vi "SJ_Enter_Data.vi"() -> (3 "SJ Data OUT":T1={"Do (mm)"=3.0, "Dc (mm)"=0.039, "Ho (mm)"=0.01, "Hc (mm)"=0.006, "K"=1.251, "beta"=1.039, "Vc (m^3)"=0.0, "Vo (m^3)"=0.0})   [LabVIEW 2011]
uses:
  Controls/SJ_Data_Cluster.ctl
panel:
  out "String":string
  in  "OK Button":bool
  in  "SJ Data IN":T1={"Do (mm)"=3.0, "Dc (mm)"=0.039, "Ho (mm)"=0.01, "Hc (mm)"=0.006, "K"=1.251, "beta"=1.039, "Vc (m^3)"=0.0, "Vo (m^3)"=0.0}
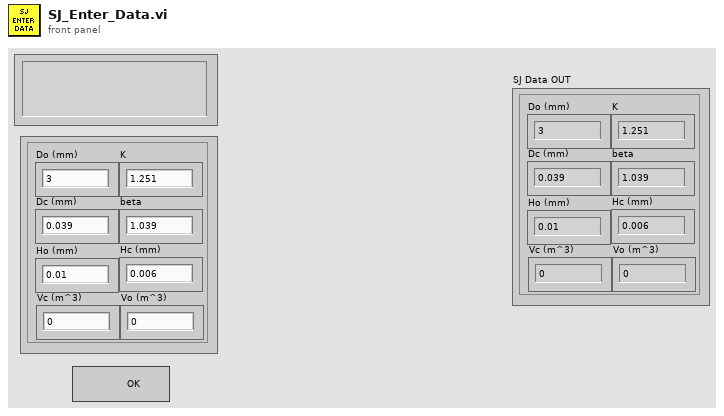
[diagram p1: front panel]
types:
  T1 = typedef "SJ_Data_Cluster.ctl" = cluster{"Do (mm)":dbl, "Dc (mm)":dbl, "Ho (mm)":dbl, "Hc (mm)":dbl, "K":dbl, "beta":dbl, "Vc (m^3)":dbl, "Vo (m^3)":dbl}
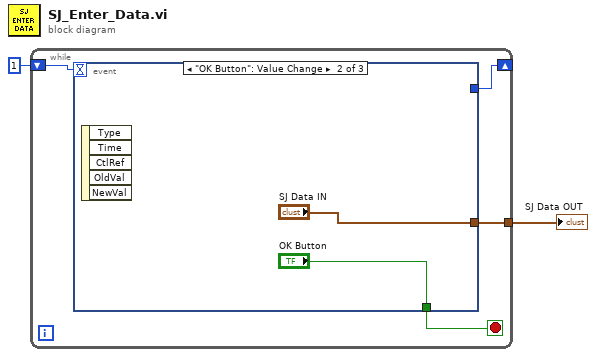
[diagram p0: block diagram]
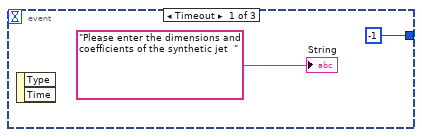
[diagram p2: hidden frame]
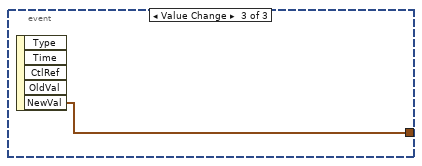
[diagram p3: hidden frame]
diagram:
  n1 = while {
    shift-right: [w5] -> _
    shift-left: 1 -> [w6]
    tunnel: [w4] -> w1
    stop <- w3 stop-if-true
    n2 = event shown="[1] \"OK Button\": Value Change" {
      selector: _ -> [_ _ _]
      dyn-events: _ -> [_ _ _]
      timeout: w6 -> [_ _ _]
      tunnel: [-1 _ _] -> w5
      tunnel: [_ "SJ Data IN" w11] -> w4
      tunnel: [_ "OK Button" _] -> w3
      event Timeout {
        n3 = event-data() -> ()  [unwired: 1 in, 2 out]
        "String" <- "Please enter the dimensions and coefficients of the synthetic jet  " ("String")
      }
      event "OK Button": Value Change {
        n4 = event-data() -> ()  [unwired: 1 in, 5 out]
      }
      event Value Change {
        n5 = event-data() -> ("NewVal"=w11:T1)  [unwired: 1 in, 4 out]
      }
    }
  }
  "SJ Data OUT" <- w1
